vi "HCC Extract Rows.vi"(7 "Station Group":T1, 8 "error in (no error)":errorcluster, 9 "String":string[](array[string]), 10 "Saving":bool[](array[boolean]), 11 "Board Index":dbl[](array[numeric])) -> (0 "error out":errorcluster, 1 "String Output":string[](array[string]), 2 "Boolean Array":bool[](array[boolean]), 3 "Board Index":dbl[](array[numeric]))   [LabVIEW 2018]
uses:
  Type Definitions/HCC Station Group.ctl
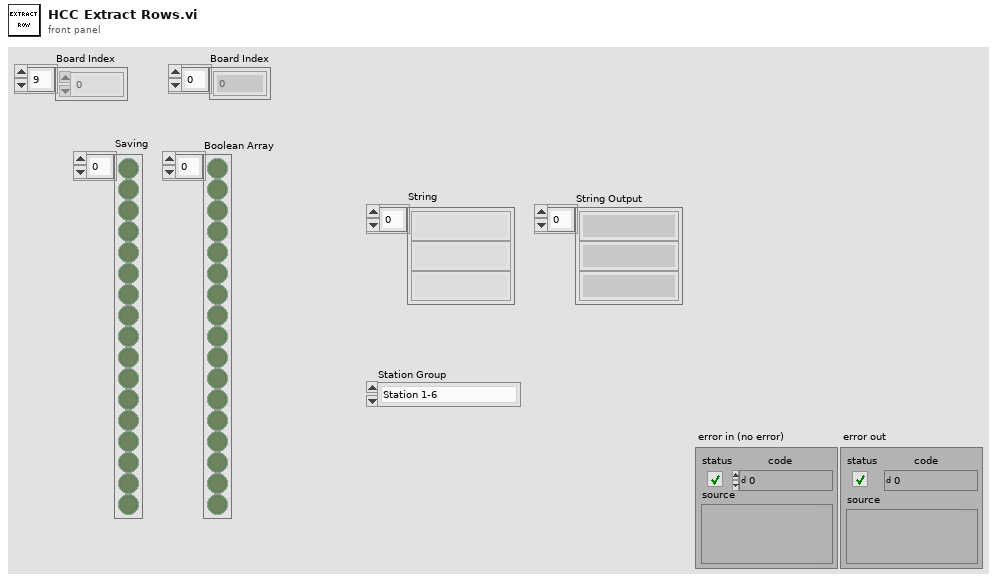
[diagram p1: front panel]
types:
  T1 = typedef "HCC Station Group.ctl" = enum16{"Station 1-6", "Station 7-12", "Station 13-18", "Station 19-24"}
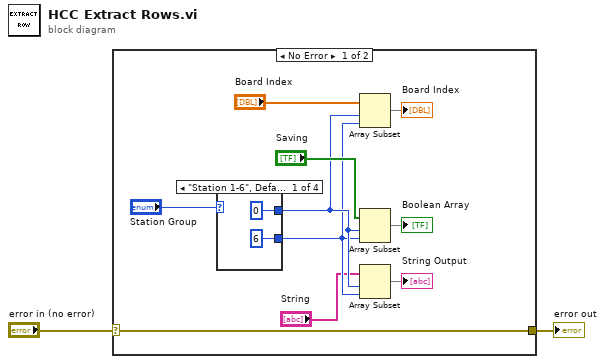
[diagram p0: block diagram]
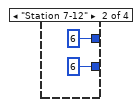
[diagram p2: hidden frame]
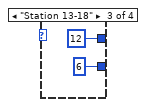
[diagram p3: hidden frame]
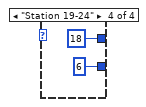
[diagram p4: hidden frame]
diagram:
  n1 = case shown="No Error" "error in (no error)" {
    selector: "error in (no error)" -> [w3 w21]
    tunnel: [w3 w21] -> w1
    frame No Error {
      n2 = case shown="\"Station 1-6\", Default" "Station Group" {
        tunnel: [0 6 12 18] -> w8
        tunnel: [6 6 6 6] -> w7
        frame "Station 1-6", Default {
        }
        frame "Station 7-12" {
        }
        frame "Station 13-18" {
        }
        frame "Station 19-24" {
        }
      }
      n3 = Array Subset(array="Board Index", index=w8, length=w7) -> (→"Board Index":dbl[])
      n4 = Array Subset(array="Saving", index=w8, length=w7) -> (→"Boolean Array":bool[])
      n5 = Array Subset(array="String", index=w8, length=w7) -> (→"String Output":string[])
    }
    frame Error {
    }
  }
  "error out" <- w1
